vi "MotorMoveAbsPos.vi"(7 "error in (no error)":errorcluster caption="错误输入（无错误）", 8 "Chan Ident":string="1", 9 "absolute position/mm":i32=10, 10 "VISA资源名称":refnum<visa-resource-name>="COM1") -> (0 "error out":errorcluster caption="错误输出", 2 "MoveCOMPLETE":bool)   [LabVIEW 2017]
uses:
  <vilib>/Instr/_visa.llb/VISA Configure Serial Port (Instr).vi
panel:
  out "res_Homed":string
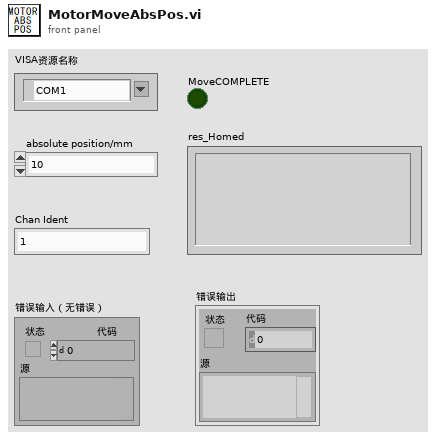
[diagram p1: front panel]
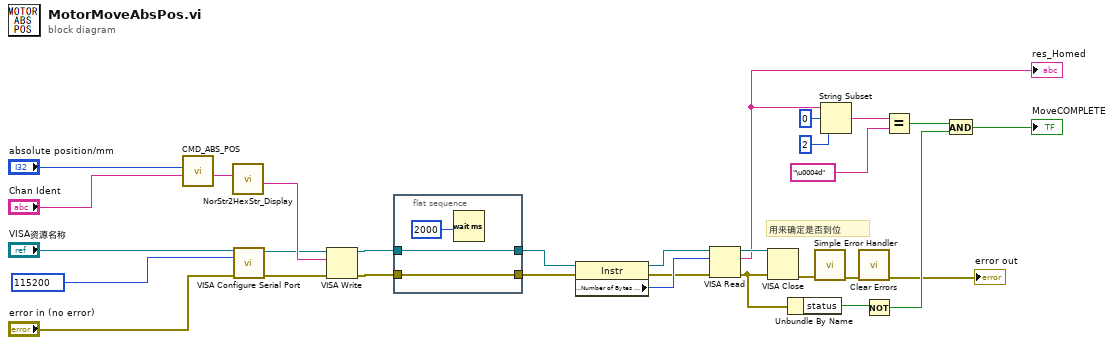
[diagram p0: block diagram]
diagram:
  w3 = u32 115200 items=["75"=75, "110"=110, "134"=134, "150"=150, "300"=300, "600"=600, "1200"=1200, "1800"=1800, "2400"=2400, "4800"=4800, "7200"=7200, "9600"=9600, "14400"=14400, "19200"=19200, "28800"=28800, "38400"=38400, "56000"=56000, "57600"=57600, "115200"=115200, "128000"=128000, "230400"=230400] ("波特率")
  # "用来确定是否到位"
  n1 = call "CMD_ABS_POS.vi"("Chan Ident"="Chan Ident", "absolute position/mm"="absolute position/mm") -> ("Command"=w7:string)  [unwired: 9 in]
  n2 = call "NorStr2HexStr_Display.vi"("Normal Display"=w7) -> ("Hex Display"=w6:string)  [unwired: 10 in]
  n3 = call-poly "VISA Configure Serial Port"("VISA resource name"="VISA资源名称", "baud rate (9600)"=w3, "error in (no error)"="error in (no error)") -> ("VISA resource name out"=w5:refnum<visa-resource-name>, "error out"=w4:errorcluster)  [unwired: 6 in, 5 out]
  n4 = VISA Write(VISA resource name=w5, write buffer=w6, error in (no error)=w4) -> (VISA resource name out=w23:refnum<visa-resource-name>, error out=w22:errorcluster)  [unwired: 1 out]
  n5 = flat-sequence {
    tunnel: w22 -> [w33]
    tunnel: [w33] -> w24
    tunnel: w23 -> [w32]
    tunnel: [w32] -> w25
    frame #0 {
      n6 = Wait (ms)(milliseconds to wait=u32 2000 ("读取前延时(ms)")) -> ()  [unwired: 1 out]
    }
  }
  n7 = property class="Instr"(reference=w25, error in=w24) -> (reference out=w26:refnum<visa-resource-name>, error out=w27:errorcluster, "Serial Settings:Number of Bytes at Serial Port"=w28:u32)
  n8 = VISA Read(VISA resource name=w26, byte count=w28, error in (no error)=w27) -> (VISA resource name out=w21:refnum<visa-resource-name>, read buffer=w16:string, error out=w15:errorcluster)  [unwired: 1 out]
  "res_Homed" <- w16
  n9 = VISA Close(VISA resource name=w21, error in (no error)=w15) -> (error out=w29:errorcluster)
  n10 = Unbundle By Name(w15) -> ("status"=w14:bool)
  n11 = call <vilib>:"Simple Error Handler.vi"("error in (no error)"=w29) -> ("error out"=w13:errorcluster)  [unwired: 1 in, 7 out]
  n12 = String Subset(string=w16, offset (0)=0 ("偏移量(0)"), length (rest)=2 ("长度（剩余）")) -> (substring=w18:string)
  n13 = call <vilib>:"Clear Errors.vi"("error in (no error)"=w13) -> ("error out"=→"error out":errorcluster)  [unwired: 5 in, 1 out]
  n14 = Not(x=w14) -> (.not. x?=w11:bool)
  n15 = Equal?(x=w18, y="\u0004d") -> (x = y?=w12:bool)
  n16 = And(x=w12, y=w11) -> (x .and. y?=→"MoveCOMPLETE":bool)
